vi "Get Controller Config.vi"(8 "error in (no error)":errorcluster, 11 "Form Model Configuration in":refnum<class "Form Model Configuration.lvclass">) -> (0 "error out":errorcluster, 2 "Controller config":refnum<class "Panel Form Controller Configuration.lvclass">, 3 "Form Model Configuration out":refnum<class "Form Model Configuration.lvclass">)   [LabVIEW 2020, in "Form Model Configuration.lvlib" / "Form Model Configuration.lvclass"]
uses:
  Form Model Configuration.lvclass
  Controller Configuration/Panel Form Controller Configuration.lvclass
  Form Model Configuration.lvclass/Form Model Configuration.ctl
  Form Controller/Panel Form Controller.lvclass/Panel Form Controller.ctl
  Form Controller/Panel Form Controller.lvclass
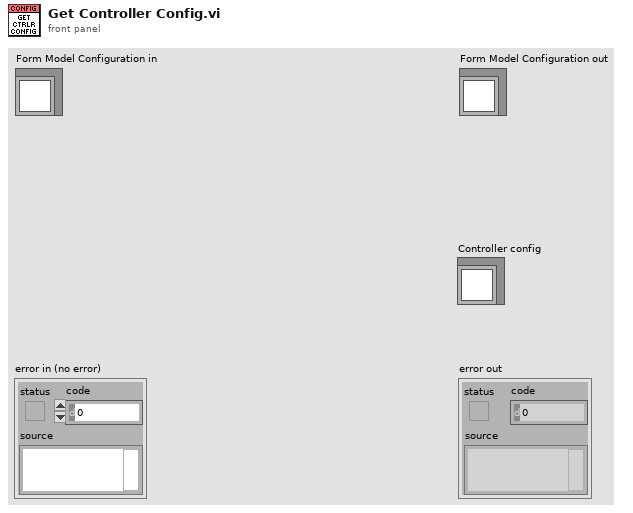
[diagram p1: front panel]
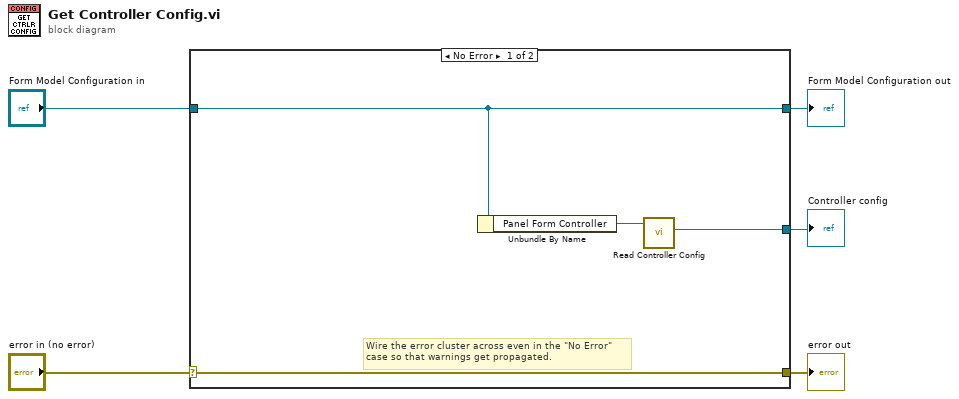
[diagram p0: block diagram]
diagram:
  n1 = case shown="No Error" "error in (no error)" {
    selector: "error in (no error)" -> [w9 w11]
    tunnel: [w9 w11] -> w4
    tunnel: [w8 w10] -> w2
    tunnel: "Form Model Configuration in" -> [w8 w10]
    tunnel: [w6 _] -> w1
    frame No Error {
      # "Wire the error cluster across even in the \"No Error\"\ncase so that warnings get propagated."
      n2 = Unbundle By Name(w8) -> ("Panel Form Controller"=w7:refnum<class "Panel Form Controller.lvclass">)
      n3 = call "Read Controller Config.vi"("Panel Form Controller in"=w7) -> ("Controller Config"=w6:refnum<class "Panel Form Controller Configuration.lvclass">)  [unwired: 8 in, 2 out]
    }
    frame Error {
    }
  }
  "error out" <- w4
  "Form Model Configuration out" <- w2
  "Controller config" <- w1
